vi "Sort_table.vi"(1 "Column":i32, 2 "Table-In":string[][](array[string])) -> (0 "Table-Out":string[][](array[string]))   [LabVIEW 2011]
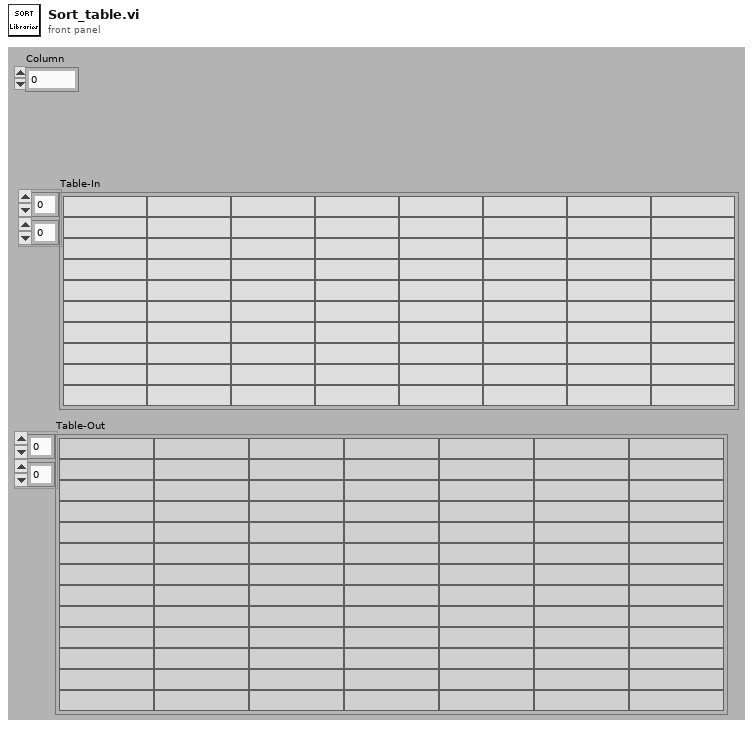
[diagram p1: front panel]
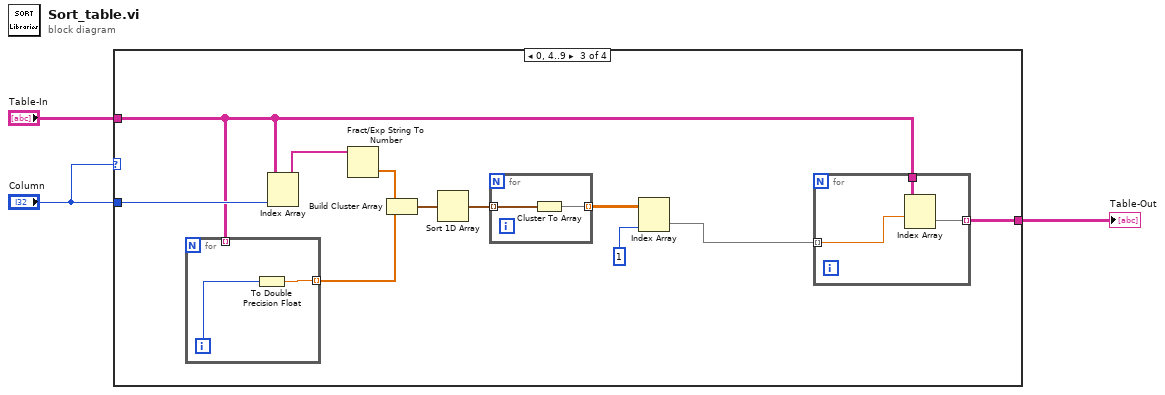
[diagram p0: block diagram]
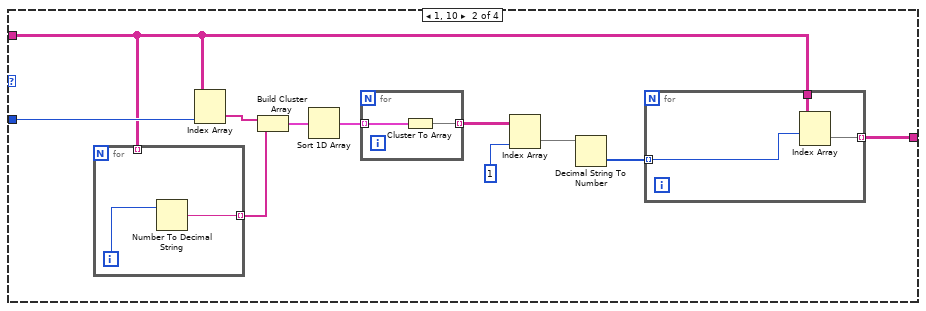
[diagram p3: hidden frame]
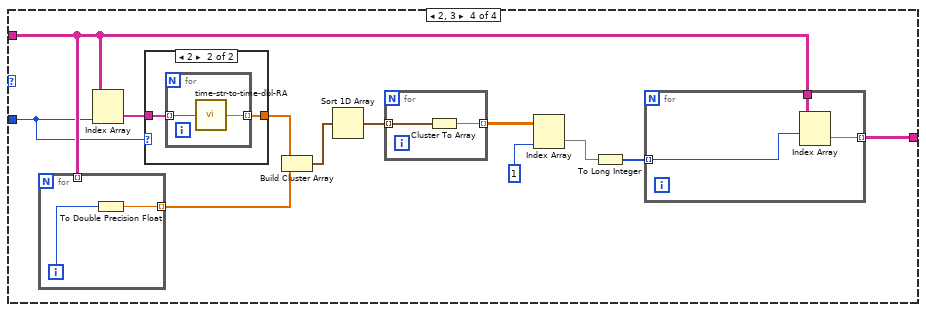
[diagram p4: hidden frame]
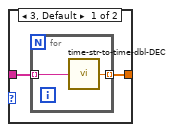
[diagram p5: hidden frame]
diagram:
  n1 = case shown="0, 4..9" "Column" {
    tunnel: "Table-In" -> [w4 w5 w24 w45]
    tunnel: [w4 w9 w30 w49] -> w2
    tunnel: "Column" -> [_ w8 w29 w44]
    frame Default {
    }
    frame 1, 10 {
      n2 = for {
        tunnel: [w16] -> w6 mode=indexing
        tunnel: w5 -> [_] mode=indexing
        i -> [w17]
        n3 = Number To Decimal String(number=w17) -> (decimal integer string=w16:string)  [unwired: 1 in]
      }
      n4 = Index Array(array=w5, index (col)=w8) -> (element=w14:string[])  [unwired: 1 in]
      n5 = Build Cluster Array(w14, w6) -> (w13:cluster{"String":string, string}[])
      n6 = Sort 1D Array(array=w13) -> (sorted array=w15:cluster{"String":string, string}[])
      n7 = for {
        tunnel: w15 -> [w22] mode=indexing
        tunnel: [w21] -> w12 mode=indexing
        n8 = Cluster To Array(cluster=w22) -> (array=w21:string[])
      }
      n9 = Index Array(array=w12, index (col)=1 ("disabled index (col)")) -> (element=w11:string[])  [unwired: 1 in]
      n10 = Decimal String To Number(string=w11) -> (number=w10:i32[])  [unwired: 2 in, 1 out]
      n11 = for {
        tunnel: w10 -> [w18] mode=indexing
        tunnel: w5 -> [w20]
        tunnel: [w19] -> w9 mode=indexing
        n12 = Index Array(array=w20, index (row)=w18) -> (element=w19:string[])  [unwired: 1 in]
      }
    }
    frame 0, 4..9 {
      n13 = for {
        tunnel: w24 -> [_] mode=indexing
        tunnel: [w34] -> w23 mode=indexing
        i -> [w35]
        n14 = To Double Precision Float(number=w35) -> (double precision float=w34:dbl)
      }
      n15 = Index Array(array=w24, index (col)=w29) -> (element=w27:string[])  [unwired: 1 in]
      n16 = Fract/Exp String To Number(string=w27) -> (number=w26:dbl[])  [unwired: 3 in, 1 out]
      n17 = Build Cluster Array(w26, w23) -> (w32:cluster{"String":dbl, dbl}[])
      n18 = Sort 1D Array(array=w32) -> (sorted array=w33:cluster{"String":dbl, dbl}[])
      n19 = for {
        tunnel: w33 -> [w40] mode=indexing
        tunnel: [w39] -> w31 mode=indexing
        n20 = Cluster To Array(cluster=w40) -> (array=w39:dbl[])
      }
      n21 = Index Array(array=w31, index (col)=1 ("disabled index (col)")) -> (element=w25:dbl[])  [unwired: 1 in]
      n22 = for {
        tunnel: w25 -> [w36] mode=indexing
        tunnel: w24 -> [w38]
        tunnel: [w37] -> w30 mode=indexing
        n23 = Index Array(array=w38, index (row)=w36) -> (element=w37:string[])  [unwired: 1 in]
      }
    }
    frame 2, 3 {
      n24 = for {
        tunnel: [w61] -> w46 mode=indexing
        tunnel: w45 -> [_] mode=indexing
        i -> [w62]
        n25 = To Double Precision Float(number=w62) -> (double precision float=w61:dbl)
      }
      n26 = Index Array(array=w45, index (col)=w44) -> (element=w43:string[])  [unwired: 1 in]
      n27 = case shown="2" w44 {
        tunnel: w43 -> [w54 w58]
        tunnel: [w53 w57] -> w42
        frame 3, Default {
          n28 = for {
            tunnel: w54 -> [w56] mode=indexing
            tunnel: [w55] -> w53 mode=indexing
            n29 = call "time-str-to-time-dbl-DEC.vi"("Chaîne"=w56) -> ("TCS_coords"=w55:dbl)
          }
        }
        frame 2 {
          n30 = for {
            tunnel: w58 -> [w60] mode=indexing
            tunnel: [w59] -> w57 mode=indexing
            n31 = call "time-str-to-time-dbl-RA.vi"("Chaîne"=w60) -> ("TCS_coords"=w59:dbl)
          }
        }
      }
      n32 = Build Cluster Array(w42, w46) -> (w51:cluster{"TCS_coords":dbl, dbl}[])
      n33 = Sort 1D Array(array=w51) -> (sorted array=w52:cluster{"TCS_coords":dbl, dbl}[])
      n34 = for {
        tunnel: w52 -> [w67] mode=indexing
        tunnel: [w66] -> w50 mode=indexing
        n35 = Cluster To Array(cluster=w67) -> (array=w66:dbl[])
      }
      n36 = Index Array(array=w50, index (col)=1 ("disabled index (col)")) -> (element=w47:dbl[])  [unwired: 1 in]
      n37 = To Long Integer(number=w47) -> (32bit integer=w41:i32[])
      n38 = for {
        tunnel: w41 -> [w63] mode=indexing
        tunnel: w45 -> [w65]
        tunnel: [w64] -> w49 mode=indexing
        n39 = Index Array(array=w65, index (row)=w63) -> (element=w64:string[])  [unwired: 1 in]
      }
    }
  }
  "Table-Out" <- w2
